vi "[GV]_IMU Port NUM.vi"() -> ()   [LabVIEW 2016]
panel:
  in  "IMU port in":refnum<visa-resource-name>="COM4"
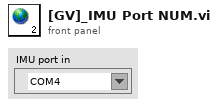
[diagram p1: front panel]
diagram:
